vi "MaxAbsScaler.vi"(8 "error in (no error)":errorcluster caption="entrée d'erreur (pas d'erreur)", 11 "MaxAbsScaler":cluster{"copy":bool}={"copy"=TRUE}) -> (0 "error out":errorcluster, 3 "MaxAbsScaler.lvclass":refnum<class "MaxAbsScaler.lvclass">)   [LabVIEW 2020]
doc: "Scale each feature by its maximum absolute value.\n\nThis estimator scales and translates each feature individually such that the maximal absolute value of each feature in the training set will be 1.0. It does not shift/center the data, and thus does not destroy any sparsity.\n\nThis scaler can also be applied to sparse CSR or CSC matrices.\n\n\nParameters : \n\n- copy : boolean, optional, default is True\nSet to False to perform inplace scaling and avoid a copy (if the input is already a numpy array).\n\n\nMethods : Compute the maximum absolute value to be used for later scaling.\n\nParameters : X : {array-like, sparse matrix}, shape [n_samples, n_features]\n The data used to compute the per-feature minimum and maximum used for later scaling along the features axis.\n\n\n- Fit Transform : Fit to data, then transform it. Fits transformer to X and y with optional parameters fit_params and returns a transformed version of X.\n\nParameters : X : {array-like, sparse matrix, dataframe} of shape (n_samples, n_features)\n y : ndarray of shape (n_samples,), default=None\n Target values.\n\nReturns : X_new : ndarray array of shape (n_samples, n_features_new)\n Transformed array.\n\n\n- Transform : Scale the data\n\nParameters : X : {array-like, sparse matrix}\n The data that should be scaled.\n\n\n- Partial Fit : Online computation of max absolute value of X for later scaling. All of X is processed as a single batch. This is intended for cases when fit is not feasible due to very large number of n_samples or because X is read from a continuous stream.\n\nParameters : X : {array-like, sparse matrix}, shape [n_samples, n_features]\n The data used to compute the mean and standard deviation used for later scaling along the features axis.\n y : None\n Ignored."
uses:
  MaxAbsScaler.lvclass
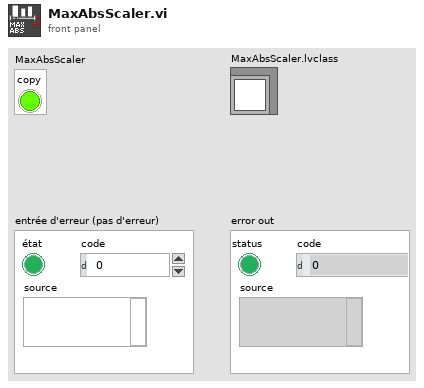
[diagram p1: front panel]
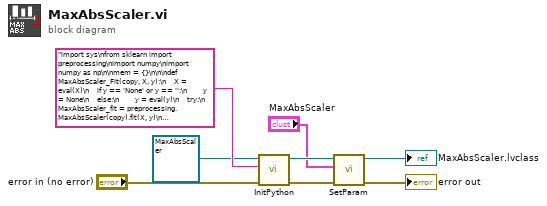
[diagram p0: block diagram]
diagram:
  n1 = call-dynamic "InitPython.vi"("error in (no error)"="error in (no error)", "Python Instruction"="import sys\nfrom sklearn import preprocessing\nimport numpy\nimport numpy as np\n\nmem = {}\n\n\ndef MaxAbsScaler_Fit(copy, X, y):\n    X = eval(X)\n    if y == 'None' or y == '':\n        y = None\n    else:\n        y = eval(y)\n    try:\n        MaxAbsScaler_fit = preprocessing.MaxAbsScaler(copy).fit(X, y)\n        mem['FitMaxAbsScaler'] = MaxAbsScaler_fit\n        return str('OK')\n    except:\n        erreur = sys.exc_info()\n        typerr = u\"%s\" % (erreur[0])\n        typerr = typerr[typerr.find(\"'\")+1:typerr.rfind(\"'\")]\n        msgerr = u\"%s\" % (erreur[1])\n        message = str('/!\\\\ {0} : {1}'. format(typerr,msgerr))\n        return message \n    \ndef MaxAbsScaler_FitTransform(copy, X, y):\n    X = eval(X)\n    if y == 'None' or y == '':\n        y = None\n    else:\n        y = eval(y)\n    try:\n        MaxAbsScaler = preprocessing.MaxAbsScaler(copy).fit_transform(X, y)\n        dtype = type(MaxAbsScaler)\n        if dtype == numpy.ndarray:\n            MaxAbsScaler = MaxAbsScaler.tolist()\n            return str(MaxAbsScaler) \n        else:\n            Mat = MaxAbsScaler.tocoo()\n            return str(list(zip(Mat.row, Mat.col, Mat.data)))\n    except:\n        erreur = sys.exc_info()\n        typerr = u\"%s\" % (erreur[0])\n        typerr = typerr[typerr.find(\"'\")+1:typerr.rfind(\"'\")]\n        msgerr = u\"%s\" % (erreur[1])\n        message = str('/!\\\\ {0} : {1}'. format(typerr,msgerr))\n        return message \n\ndef MaxAbsScaler_Transform(copy, X, y):\n    X = eval(X)\n    if y == 'None' or y == '':\n        y = None\n    else:\n        y = eval(y)\n    try:\n        MaxAbsScaler = mem['FitMaxAbsScaler'].transform(X)\n        dtype = type(MaxAbsScaler)\n        if dtype == numpy.ndarray:\n            MaxAbsScaler = MaxAbsScaler.tolist()\n            return str(MaxAbsScaler) \n        else:\n            Mat = MaxAbsScaler.tocoo()\n            return str(list(zip(Mat.row, Mat.col, Mat.data)))\n    except:\n        erreur = sys.exc_info()\n        typerr = u\"%s\" % (erreur[0])\n        typerr = typerr[typerr.find(\"'\")+1:typerr.rfind(\"'\")]\n        msgerr = u\"%s\" % (erreur[1])\n        message = str('/!\\\\ {0} : {1}'. format(typerr,msgerr))\n        return message\n    \ndef MaxAbsScaler_Partial_Fit(copy, X, y):\n    X = eval(X)\n    if y == 'None' or y == '':\n        y = None\n    else:\n        y = eval(y)\n    try:\n        MaxAbsScaler = preprocessing.MaxAbsScaler(copy).partial_fit(X, y)\n        mem['FitMaxAbsScaler'] = MaxAbsScaler\n        return str('OK')\n    except:\n        erreur = sys.exc_info()\n        typerr = u\"%s\" % (erreur[0])\n        typerr = typerr[typerr.find(\"'\")+1:typerr.rfind(\"'\")]\n        msgerr = u\"%s\" % (erreur[1])\n        message = str('/!\\\\ {0} : {1}'. format(typerr,msgerr))\n        return message", "Scikit-learn en entrée"=refnum<class "MaxAbsScaler.lvclass"> refnum ("MaxAbsScaler.lvclass")) -> ("error out"=w4:errorcluster, "Scikit-learn en sortie"=w5:refnum<class "MaxAbsScaler.lvclass">)  [unwired: 7 in]
  n2 = call-dynamic "SetParam.vi"("error in (no error)"=w4, "MaxAbsScaler"="MaxAbsScaler", "MaxAbsScaler.lvclass"=w5) -> ("error out"=→"error out":errorcluster, "MaxAbsScaler.lvclass"=→"MaxAbsScaler.lvclass":refnum<class "MaxAbsScaler.lvclass">)  [unwired: 7 in]
